vi "Test_stage.vi"() -> ()   [LabVIEW 2018]
uses:
  C:/Project/SerialSectOCT/Labview Software/Thorlabs.MotionControl.Controls.dll
  Thorlabs.MotionControl.Controls.dll
  C:/Project/SerialSectOCT/Labview Software/Thorlabs.MotionControl.IntegratedStepperMotorsCLI.dll
  Thorlabs.MotionControl.IntegratedStepperMotorsCLI.dll
panel:
  in  "Y LongTravelStageControl":refnum<k24>(container)
  in  "Stages":T1={"X LTS Serial No."="", "Y LTS Serial No."="", "Z MLJ Serial No."="", "To Cut maxVelocity"=0.0, "To Cut acceleration"=0.0, "X Start position"=5.0, "Timeout"=0, "Cut Length"=5.0, "Cut maxVelocity"=0.0, "Cut acceleration"=0.0, "Y Start position"=5.0, "Z maxVelocity"=0.0, "Z acceleration"=0.0, "Z Move position"=5.0, "Z Cut position"=5.0, "Cut Direction"=""} {"Z Cut position" min=0.0 max=150.0 format="%#_13g"; "Z Move position" min=0.0 max=150.0 format="%#_13g"; "Y Start position" min=0.0 max=150.0 format="%#_13g"; "Cut Length" min=0.0 max=150.0 format="%#_13g"; "X Start position" min=0.0 max=150.0 format="%#_13g"}
  in  "X LongTravelStageControl":refnum<k24>(container)
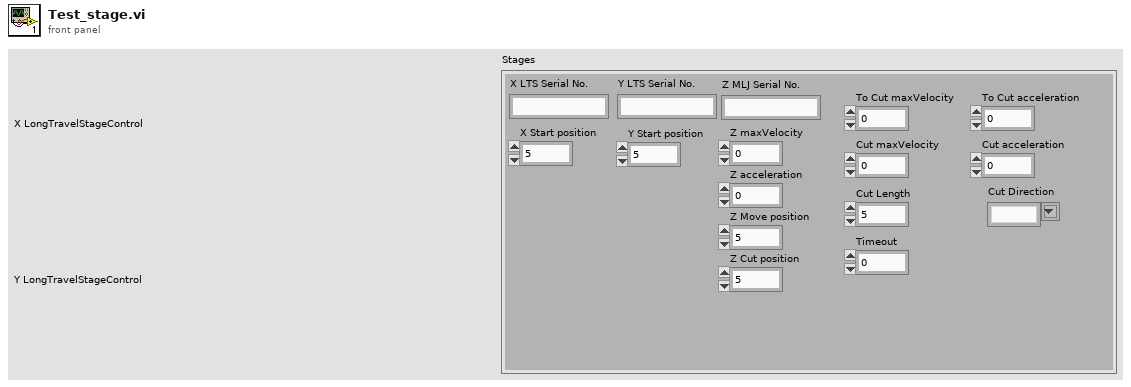
[diagram p1: front panel]
types:
  T1 = cluster{"X LTS Serial No.":string, "Y LTS Serial No.":string, "Z MLJ Serial No.":string, "To Cut maxVelocity":dbl, "To Cut acceleration":dbl, "X Start position":dbl, "Timeout":i32, "Cut Length":dbl, "Cut maxVelocity":dbl, "Cut acceleration":dbl, "Y Start position":dbl, "Z maxVelocity":dbl, "Z acceleration":dbl, "Z Move position":dbl, "Z Cut position":dbl, "Cut Direction":string}
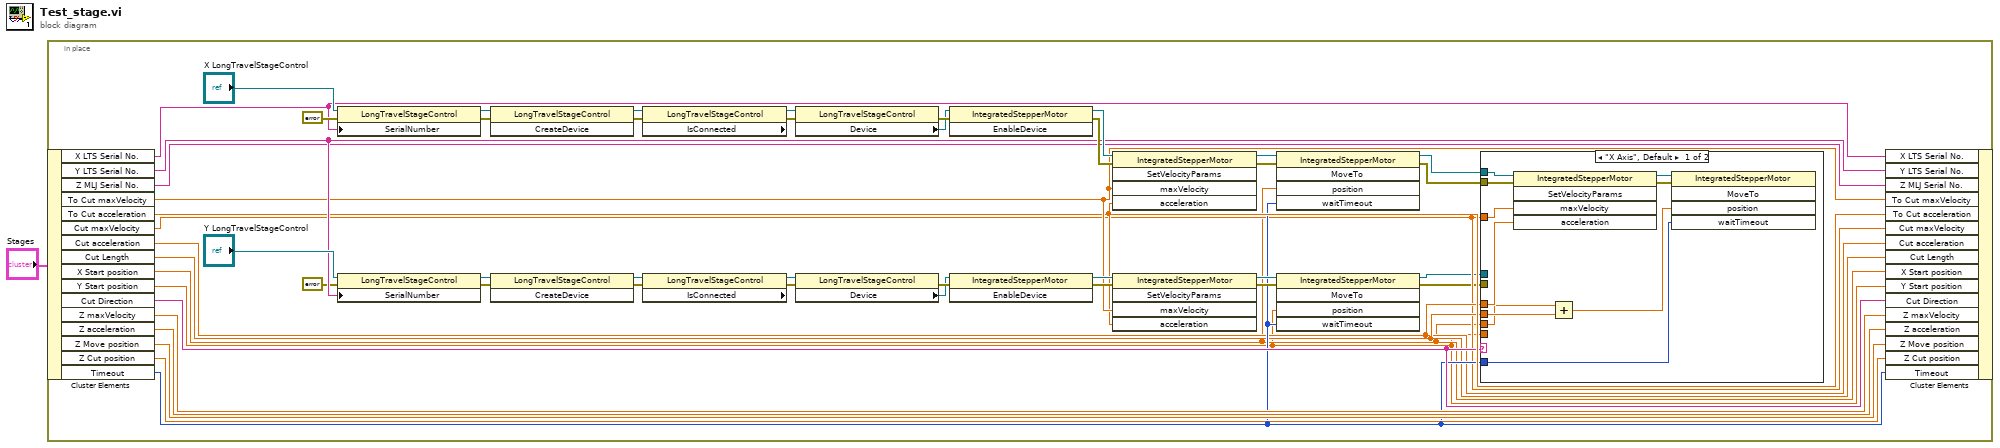
[diagram p0: block diagram]
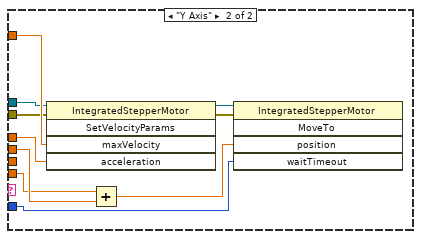
[diagram p2: hidden frame]
diagram:
  n1 = in-place {
    n2 = in-place-cluster #1("Stages") -> ("X LTS Serial No."=w24:string, "Y LTS Serial No."=w23:string, "Z MLJ Serial No."=w18:string, "To Cut maxVelocity"=w13:dbl, "To Cut acceleration"=w12:dbl, "Cut maxVelocity"=w7:dbl, "Cut acceleration"=w8:dbl, "Cut Length"=w9:dbl, "X Start position"=w6:dbl, "Y Start position"=w5:dbl, "Cut Direction"=w11:string, "Z maxVelocity"=w17:dbl, "Z acceleration"=w16:dbl, "Z Move position"=w15:dbl, "Z Cut position"=w14:dbl, "Timeout"=w10:i32)
    n3 = property class="LongTravelStageControl"(reference="X LongTravelStageControl", error in=errorcluster {"status"=FALSE, "code"=0, "source"=""} ("error in (no error)"), "SerialNumber"=w24) -> (reference out=w47:refnum<k24>, error out=w44:errorcluster)
    n4 = property class="LongTravelStageControl"(reference="Y LongTravelStageControl", error in=errorcluster {"status"=FALSE, "code"=0, "source"=""} ("error in (no error)"), "SerialNumber"=w23) -> (reference out=w35:refnum<k24>, error out=w32:errorcluster)
    n5 = invoke class="LongTravelStageControl" method="CreateDevice"(reference=w47, error in=w44) -> (reference out=w46:refnum<k24>, error out=w45:errorcluster)  [unwired: 1 in, 1 out]
    n6 = invoke class="LongTravelStageControl" method="CreateDevice"(reference=w35, error in=w32) -> (reference out=w34:refnum<k24>, error out=w33:errorcluster)  [unwired: 1 in, 1 out]
    n7 = property class="LongTravelStageControl" props=["IsConnected"](reference=w46, error in=w45) -> (reference out=w43:refnum<k24>, error out=w42:errorcluster)  [unwired: 1 out]
    n8 = property class="LongTravelStageControl" props=["IsConnected"](reference=w34, error in=w33) -> (reference out=w31:refnum<k24>, error out=w30:errorcluster)  [unwired: 1 out]
    n9 = property class="LongTravelStageControl"(reference=w43, error in=w42) -> (error out=w41:errorcluster, "Device"=w40:refnum<k24>)  [unwired: 1 out]
    n10 = property class="LongTravelStageControl"(reference=w31, error in=w30) -> (error out=w29:errorcluster, "Device"=w28:refnum<k24>)  [unwired: 1 out]
    n11 = invoke class="IntegratedStepperMotor" method="EnableDevice"(reference=w40, error in=w41) -> (reference out=w39:refnum<k24>, error out=w38:errorcluster)  [unwired: 1 in, 1 out]
    n12 = invoke class="IntegratedStepperMotor" method="EnableDevice"(reference=w28, error in=w29) -> (reference out=w27:refnum<k24>, error out=w26:errorcluster)  [unwired: 1 in, 1 out]
    n13 = invoke class="IntegratedStepperMotor" method="SetVelocityParams"(reference=w39, error in=w38, "maxVelocity"=w13, "acceleration"=w12) -> (reference out=w22:refnum<k24>, error out=w21:errorcluster)  [unwired: 1 in, 3 out]
    n14 = invoke class="IntegratedStepperMotor" method="SetVelocityParams"(reference=w27, error in=w26, "maxVelocity"=w13, "acceleration"=w12) -> (reference out=w20:refnum<k24>, error out=w19:errorcluster)  [unwired: 1 in, 3 out]
    n15 = invoke class="IntegratedStepperMotor" method="MoveTo"(reference=w22, error in=w21, "position"=w6, "waitTimeout"=w10) -> (reference out=w36:refnum<k24>, error out=w37:errorcluster)  [unwired: 1 in, 3 out]
    n16 = invoke class="IntegratedStepperMotor" method="MoveTo"(reference=w20, error in=w19, "position"=w5, "waitTimeout"=w10) -> (reference out=w4:refnum<k24>, error out=w3:errorcluster)  [unwired: 1 in, 3 out]
    n17 = case shown="\"X Axis\", Default" w11 {
      tunnel: w37 -> [w59 _]
      tunnel: w36 -> [w58 _]
      tunnel: w10 -> [w54 w66]
      tunnel: w9 -> [w53 w65]
      tunnel: w8 -> [w52 w64]
      tunnel: w7 -> [w51 w63]
      tunnel: w6 -> [w50 _]
      tunnel: w5 -> [_ w62]
      tunnel: w4 -> [_ w61]
      tunnel: w3 -> [_ w60]
      frame "X Axis", Default {
        n18 = invoke class="IntegratedStepperMotor" method="SetVelocityParams"(reference=w58, error in=w59, "maxVelocity"=w51, "acceleration"=w52) -> (reference out=w57:refnum<k24>, error out=w56:errorcluster)  [unwired: 1 in, 3 out]
        n19 = Add(x=w50, y=w53) -> (x+y=w55:dbl)
        n20 = invoke class="IntegratedStepperMotor" method="MoveTo"(reference=w57, error in=w56, "position"=w55, "waitTimeout"=w54) -> ()  [unwired: 1 in, 5 out]
      }
      frame "Y Axis" {
        n21 = invoke class="IntegratedStepperMotor" method="SetVelocityParams"(reference=w61, error in=w60, "maxVelocity"=w63, "acceleration"=w64) -> (reference out=w69:refnum<k24>, error out=w68:errorcluster)  [unwired: 1 in, 3 out]
        n22 = Add(x=w62, y=w65) -> (x+y=w67:dbl)
        n23 = invoke class="IntegratedStepperMotor" method="MoveTo"(reference=w69, error in=w68, "position"=w67, "waitTimeout"=w66) -> ()  [unwired: 1 in, 5 out]
      }
    }
    n24 = in-place-cluster #1("X LTS Serial No."=w24, "Y LTS Serial No."=w23, "Z MLJ Serial No."=w18, "To Cut maxVelocity"=w13, "To Cut acceleration"=w12, "Cut maxVelocity"=w7, "Cut acceleration"=w8, "Cut Length"=w9, "X Start position"=w6, "Y Start position"=w5, "Cut Direction"=w11, "Z maxVelocity"=w17, "Z acceleration"=w16, "Z Move position"=w15, "Z Cut position"=w14, "Timeout"=w10) -> ()  [unwired: 1 out]
  }
